vi "automatic_complete_continue.vi"(5 "change_in_event":refnum<user-event>, 7 "waitgroup":T1, 8 "error in (no error)":errorcluster, 11 "data":variant) -> (0 "error out":errorcluster)   [LabVIEW 2015, in "example_01.lvlib"]
uses:
  example_01.lvlib
  <userlib>/antonio-alexander/lv-waitgroup/public/_controls/api_waitgroup.ctl
  lv-recipe-machine/public/_controls/change.ctl
  lv-recipe-machine/lv-recipe-machine.lvlib
  <userlib>/antonio-alexander/lv-waitgroup/lv-waitgroup.lvlib
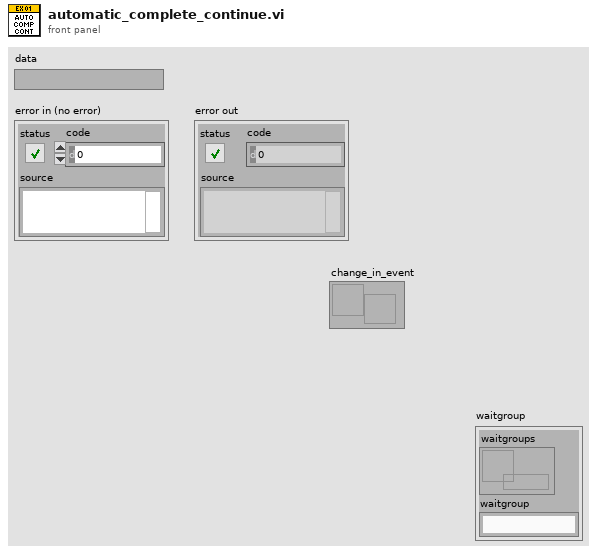
[diagram p1: front panel]
types:
  T1 = typedef "lv-waitgroup.lvlib/api_waitgroup.ctl" = cluster{"waitgroups":refnum<data-value>, "waitgroup":string}
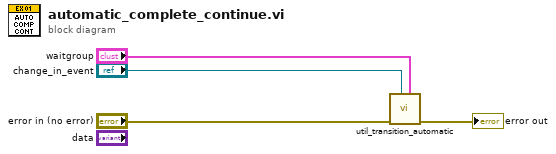
[diagram p0: block diagram]
diagram:
  n1 = call "util_transition_automatic.vi"("api_waitgroup"="waitgroup", "change_in_event"="change_in_event", "error in (no error)"="error in (no error)") -> ("error out"=→"error out":errorcluster)  [unwired: 8 in]
